vi "CalculateModeTimeRemaining.vi"(1 "StepTime":dbl[unit], 2 "StrtTime":timestamp, 3 "CurrentTime":timestamp) -> (0 "TimeRem":timestamp)   [LabVIEW 2018]
doc: "Given an input time and a start time, this VI calculates the Time Remaining for a given Step Time\n\nCopyright © 2011 Epimedia, Inc. All Rights Reserved.\n\nThe Epimedia Application Library is Copyright © 2009-2011 Epimedia, Inc. \nAll Rights Reserved. Used under license."
panel:
  # "Copyright © 2011 Epimedia, Inc. All Rights Reserved.\n\nThe Epimedia Application Library is Copyright © 2009-2011 Epimedia, Inc. \nAll Rights Reserved. Used under license."
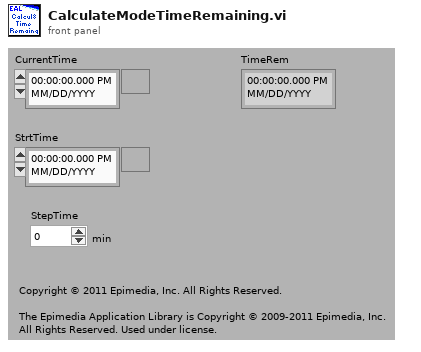
[diagram p1: front panel]
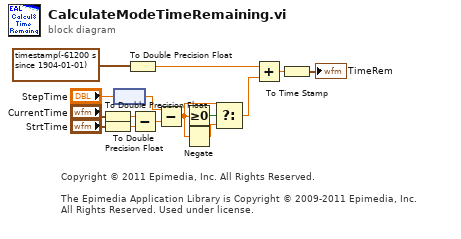
[diagram p0: block diagram]
diagram:
  # "Copyright © 2011 Epimedia, Inc. All Rights Reserved.\n\nThe Epimedia Application Library is Copyright © 2009-2011 Epimedia, Inc. \nAll Rights Reserved. Used under license."
  n1 = To Double Precision Float(number="CurrentTime") -> (double precision float=w10:dbl)
  n2 = To Double Precision Float(number="StrtTime") -> (double precision float=w11:dbl)
  n3 = node("StepTime") -> (w1:dbl)
  n4 = To Double Precision Float(number=timestamp(-61200 s since 1904-01-01) ("time stamp")) -> (double precision float=w9:dbl)
  n5 = Subtract(x=w10, y=w11) -> (x-y=w12:dbl)
  n6 = Subtract(x=w1, y=w12) -> (x-y=w5:dbl)
  n7 = Greater Or Equal To 0?(x=w5) -> (x >= 0?=w6:bool)
  n8 = Negate(x=w5) -> (-x=w4:dbl)
  n9 = Select(t=w5, s=w6, f=w4) -> (s? t:f=w3:dbl)
  n10 = Add(x=w9, y=w3) -> (x+y=w7:dbl)
  n11 = To Time Stamp(1:w7) -> (0:→"TimeRem":timestamp)
